vi "Set Waveform Type.vi"(8 "error in (no error)":errorcluster, 9 "2nd Waveform (0: None)":u32(ring) items=["None", "Sine", "Triangle", "Square", "Truncated Sine"], 10 "1st Waveform (0: None)":u32(ring) items=["None", "Sine", "Triangle", "Square", "Truncated Sine"], 11 "VISA resource name":refnum<visa-resource-name>) -> (0 "error out":errorcluster, 3 "VISA resource name out":refnum<visa-resource-name>)   [LabVIEW 2013, in "Fluke 5XXX Series Multicalibrators.lvlib"]
doc: "This VI sets the waveforms for ac outputs. If the Calibrator is sourcing one output, one parameter is required. If the Calibrator is sourcing two outputs, two parameters are required or one parameter to set the waveform to both outputs. Waveform choices are SINE (sinewave), TRI (trianglewave), SQUARE (squarewave), TRUNCS (truncated sinewave), or NONE (waveform does not apply).\n\nNote:\n\nThis VI is available only for instrument models 5500A and 5520A."
uses:
  Fluke 5XXX Series Multicalibrators.lvlib
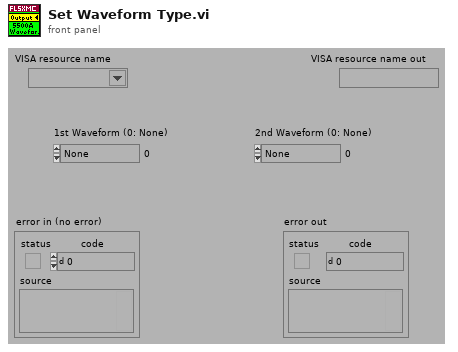
[diagram p1: front panel]
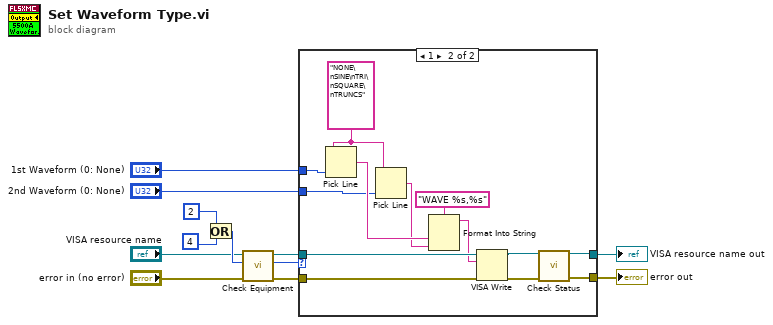
[diagram p0: block diagram]
diagram:
  n1 = Or(x=2 ("Numeric"), y=4 ("Numeric")) -> (x .or. y?=w9:i32)
  n2 = call "Check Equipment.vi"("error in (no error)"="error in (no error)", "Bit Mask"=w9, "VISA resource name"="VISA resource name") -> ("error out"=w12:errorcluster, "Present?"=w11:u32, "VISA resource name out"=w10:refnum<visa-resource-name>)  [unwired: 6 in]
  n3 = case shown="1" w11 {
    tunnel: [w13 w22] -> w5
    tunnel: w12 -> [w14 w27]
    tunnel: w10 -> [w13 w26]
    tunnel: [w14 w25] -> w6
    tunnel: "1st Waveform (0: None)" -> [_ w17]
    tunnel: "2nd Waveform (0: None)" -> [_ w16]
    frame 0, Default {
    }
    frame 1 {
      w15 = "NONE\nSINE\nTRI\nSQUARE\nTRUNCS"
      n4 = Pick Line(multi-line string=w15, line index=w17) -> (output string=w19:string)  [unwired: 1 in]
      n5 = Pick Line(multi-line string=w15, line index=w16) -> (output string=w18:string)  [unwired: 1 in]
      n6 = Format Into String(format string="WAVE %s,%s", w19, w18) -> (resulting string=w20:string)  [unwired: 2 in, 1 out]
      n7 = VISA Write(VISA resource name=w26, write buffer=w20, error in (no error)=w27) -> (VISA resource name out=w23:refnum<visa-resource-name>, error out=w24:errorcluster)  [unwired: 1 out]
      n8 = call "Check Status.vi"("VISA resource name"=w23, "error in (no error)"=w24) -> ("VISA resource name out"=w22:refnum<visa-resource-name>, "error out"=w25:errorcluster)  [unwired: 12 in]
    }
  }
  "VISA resource name out" <- w5
  "error out" <- w6
